vi "SendOracleRequest(SubVI).vi"(7 "HTTP string":string="http://force.natinst.com:8000/pls/ebiz/nic_sr_report.receive_parameters?p_email_address=denis.stavila%40ni.com&p_ae_group=100000045&p_ae_group=100000050&p_ae_group=100000059&p_ae_group=100000062&p_ae_group=100000064&p_creation_date_start=01-JAN-17&p_creation_date_end=08-JUN-17&p_sr_initiation_type=", 8 "error in (no error)":errorcluster, 9 "Timeout":i32=5000, 10 "Use current Date":bool=TRUE, 11 "Report End Date":timestamp) -> (0 "error out":errorcluster, 3 "Request ID":string)   [LabVIEW 2018, in "MainFrameLib.lvlib"]
uses:
  MainFrameLib.lvlib
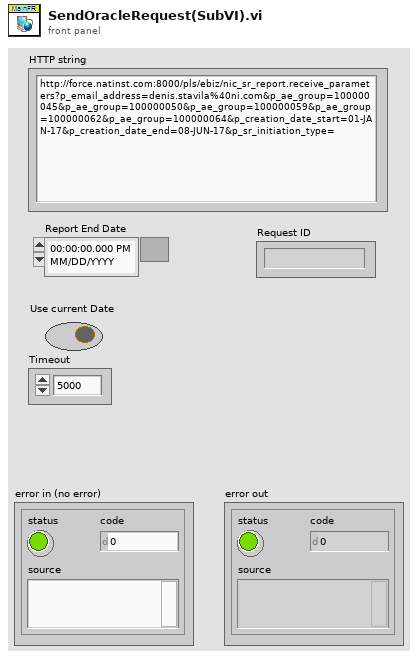
[diagram p1: front panel]
types:
  T1 = enum16{"Read", "Write", "ReadWrite", "BufferedRead", "BufferedReadWrite"}
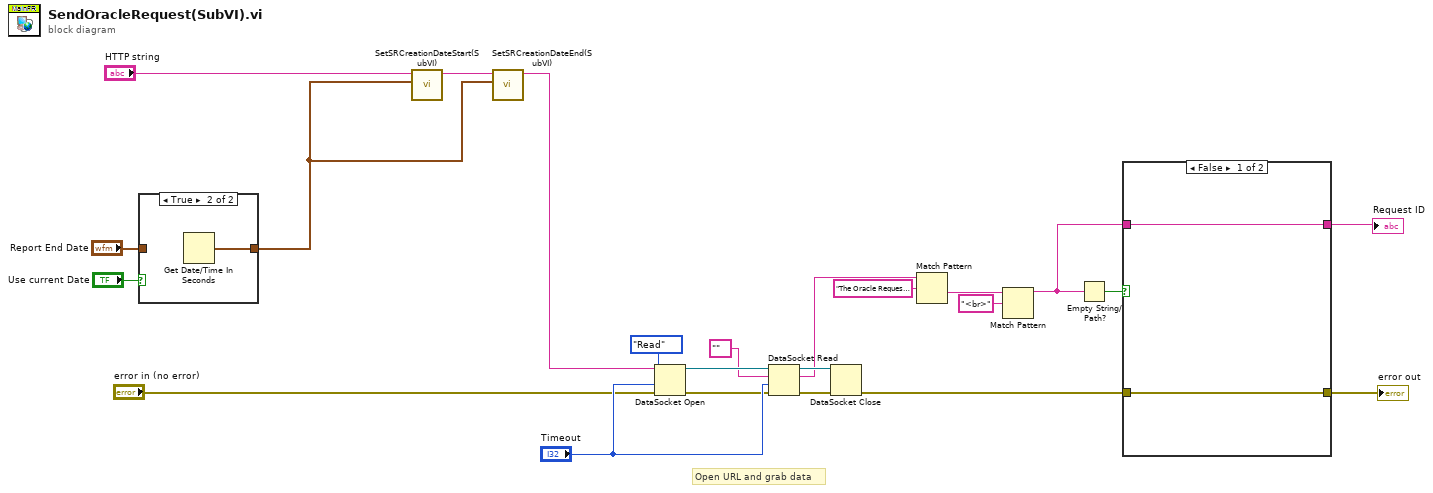
[diagram p0: block diagram]
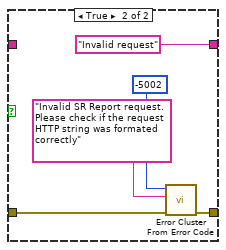
[diagram p2: hidden frame]
diagram:
  # "Open URL and grab data"
  n1 = case shown="True" "Use current Date" {
    tunnel: [w24 w25] -> w7
    tunnel: "Report End Date" -> [w24 _]
    frame False {
    }
    frame True {
      n2 = Get Date/Time In Seconds() -> (seconds since 1Jan1904=w25:timestamp)
    }
  }
  n3 = call "SetSRCreationDateStart(SubVI).vi"("Date"=w7, "HTTP string"="HTTP string") -> ("result string"=w5:string)  [unwired: 9 in]
  n4 = call "SetSRCreationDateEnd(SubVI).vi"("seconds since 1Jan1904"=w7, "HTTP string in"=w5) -> ("String"=w15:string)  [unwired: 9 in]
  n5 = DataSocket Open(8:"error in (no error)", 9:"Timeout", 10:T1."Read" ("mode"), 11:w15) -> (0:w18:errorcluster, 3:w19:refnum<k13>)
  n6 = DataSocket Read(8:w18, 9:"Timeout", 10:"", 11:w19) -> (0:w20:errorcluster, 2:w11:string, 3:w21:refnum<k13>)  [unwired: 1 in, 4 out]
  n7 = DataSocket Close(8:w20, 11:w21) -> (0:w2:errorcluster)  [unwired: 1 in, 1 out]
  n8 = Match Pattern(string=w11, regular expression="The Oracle Request ID for your report is ") -> (after substring=w13:string)  [unwired: 1 in, 3 out]
  n9 = Match Pattern(string=w13, regular expression="<br>") -> (before substring=w4:string)  [unwired: 1 in, 3 out]
  n10 = Empty String/Path?(string/path=w4) -> (empty?=w6:bool)
  n11 = case shown="False" w6 {
    tunnel: w4 -> [w27 _]
    tunnel: [w27 "Invalid request"] -> w3
    tunnel: w2 -> [w26 w31]
    tunnel: [w26 w29] -> w1
    frame False {
    }
    frame True {
      n12 = call <vilib>:"Error Cluster From Error Code.vi"("error in (no error)"=w31, "error message (\"\")"="Invalid SR Report request. Please check if the request HTTP string was formated correctly" ("error message (\"\")"), "error code (0)"=-5002) -> ("error out"=w29:errorcluster)  [unwired: 6 in]
    }
  }
  "error out" <- w1
  "Request ID" <- w3
